vi "Lap Statistics.vi"   [LabVIEW 2014]
uses:
  <vilib>/Platform/TimedLoop/XDataNode/timing_clust.ctl
  <vilib>/Platform/TimedLoop/XDataNode/nitl_modes.ctl
  <vilib>/Platform/TimedLoop/XDataNode/wakeup.ctl
  Lap Statistics.ctl
  <vilib>/FPGAPlugInAG/sbRIO-9626/niLvFpga_Open_sbRIO-9626.vi
  <vilib>/rvi/interface/common/dynamic/niFpgaDynamicAddResources.vi
  Formula Hybrid 2012 r1/Global Data.vi
  <vilib>/Utility/error.llb/Error Cluster From Error Code.vi
  <vilib>/rvi/errors/niLvFpgaAdjustHostInterfaceError.vi
  <vilib>/Platform/TimedLoop/XDataNode/XDataNode.xnode
  <vilib>/rvi/interface/nirviOpenFPGA/nirviOpenFPGA.xnode
  FPGA Bitfiles/FormulaElectric2_FPGATarget_FPGA_8a5J0mMac2U.lvbitx
  <vilib>/rvi/interface/nirviReadWriteControl/nirviReadWriteControl.xnode
  <vilib>/Platform/TimedLoop/XDataNode/XDNodeRunTimeDep.lvlib
  NiFpgaLv.dll
  <vilib>/rvi/interface/Simulation/niFpgaSimulationCallBeginRW.vi
types:
  T1 = typedef "XDNodeRunTimeDep.lvlib/timing_clust.ctl" = cluster{"Expected End [f-1]":u64, "Actual End [f-1]":u64, "Finished Late? [f-1]":bool, "Expected End [i-1]":u64, "Actual End [i-1]":u64, "Finished Late? [i-1]":bool, "Expected Start [i]":u64, "Actual Start [i]":u64, "Expected Start [f]":u64, "Actual Start [f]":u64, "Source Name":string, "Structure Name":string, "Period":i64, "Deadline":i64, "Offset":i64, "Start":i64, "Priority":i32, "Timeout":i32, "Mode":T2, "Wakeup Reason":T3, "Error":errorcluster, "Source Type":string, "Secondary Source Type":string, "Global End Time":u64, "Global Start Time":u64, "Frame Duration":u64, "Iteration Duration":u64, "Assigned CPU":i32, "I/O Scan Engine Mode":u32}
  T2 = typedef "XDNodeRunTimeDep.lvlib/nitl_modes.ctl" = enum32{"No Change", "Process missed periods, maintain original phase", "Discard missed periods, maintain original phase", "Process missed periods, ignore original phase", "Discard missed periods, ignore original phase"}
  T3 = typedef "XDNodeRunTimeDep.lvlib/wakeup.ctl" = enum32{"Normal", "Aborted", "Asynchronous wakeup", "Timing source error", "Timed loop error", "Timeout"}
  T4 = typedef "Lap Statistics.ctl" = cluster{"rBrakeBalLast":dbl}
  T5 = cluster{"Accel X":dbl, "Accel Y":dbl, "Accel Z":dbl, "Gyro X":dbl, "Gyro Y":dbl, "Gyro Z":dbl}
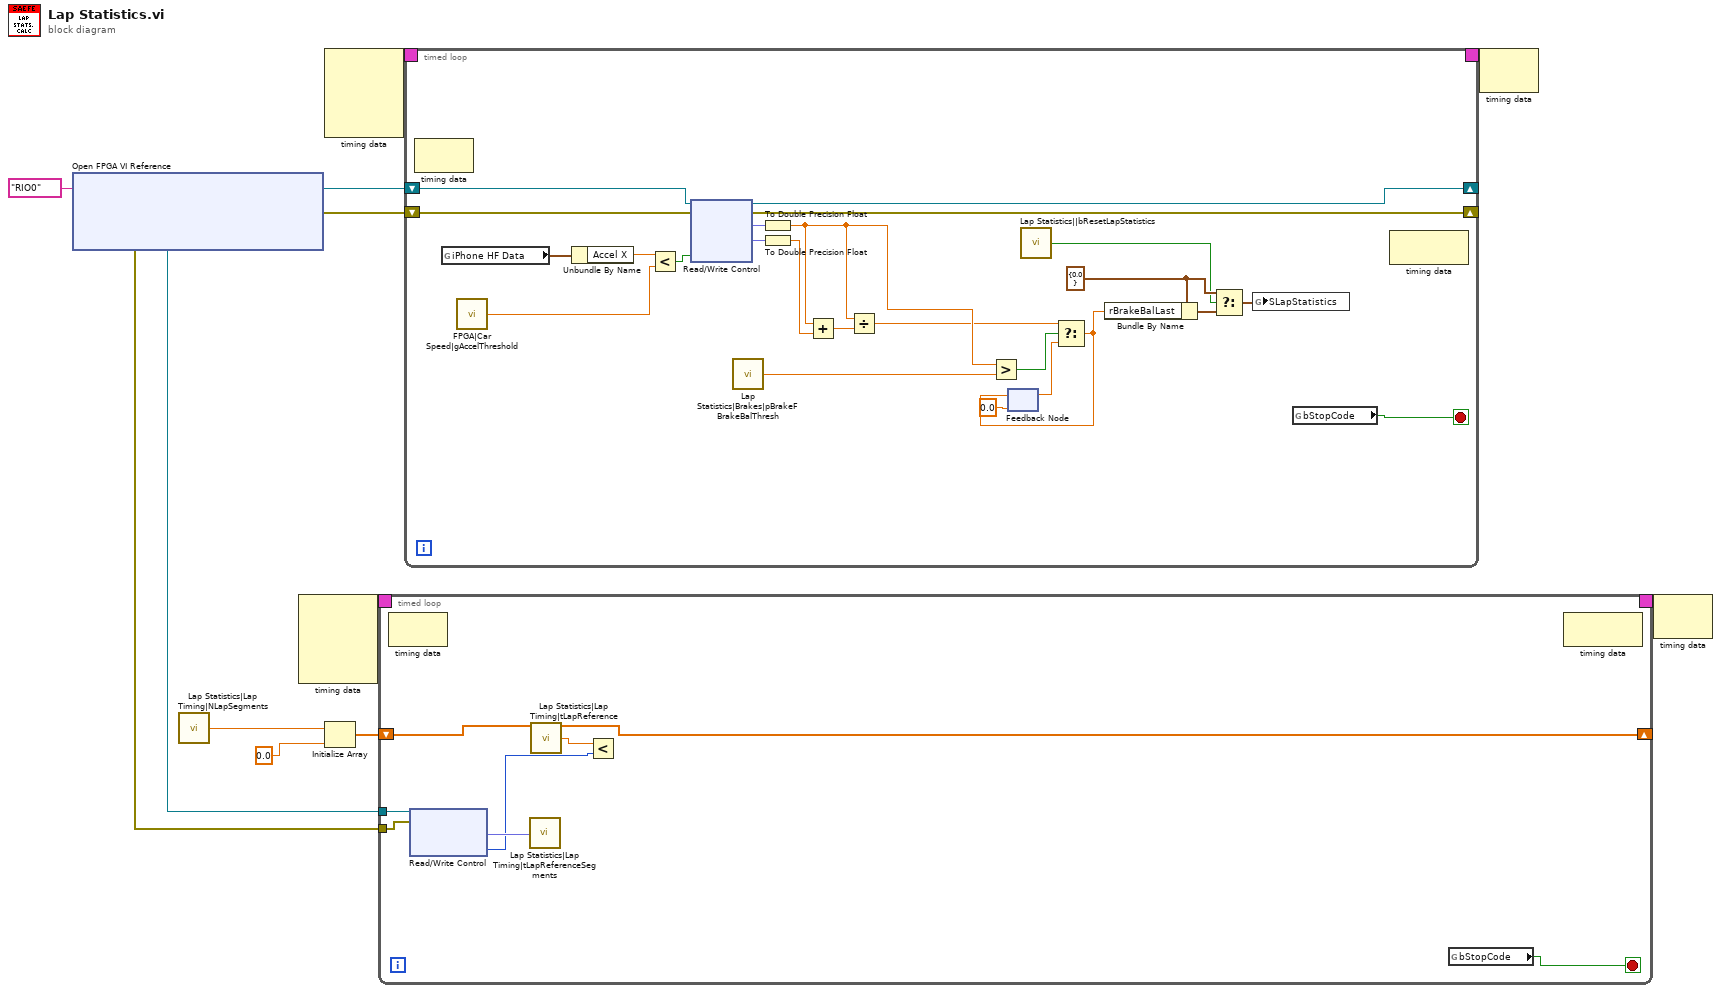
[diagram p0: block diagram]
diagram:
  n1 = xnode "Open FPGA VI Reference"("resource name"=tag "RIO0") -> ("FPGA VI Reference Out"=w5:refnum<k20>, "error out"=w4:errorcluster)  [unwired: 1 in]
  n2 = call "Lap Statistics|Lap Timing|NLapSegments"() -> ("Value"=w3:sgl)
  n3 = node-c288() -> (w7:T1)  [unwired: 4 in]
  n4 = node-c288() -> (w10:T1)  [unwired: 4 in]
  n5 = Initialize Array(w3, sgl 0.0) -> (w2:sgl[])
  n6 = timed-loop {
    timing: w7 -> [_]
    timing-out: [_] -> w6
    tunnel: w5 -> [w15]
    tunnel: w4 -> [w16]
    shift-right: [w11] -> _
    shift-left: w2 -> [w11]
    stop <- w17 stop-if-true
    n7 = node-c288() -> ()  [unwired: 1 in, 1 out]
    n8 = xnode "Read/Write Control"("FPGA VI Reference In"=w15, "error in"=w16) -> ("sLap"=w14:fxp<+,32,12>, "tFastestLap"=w12:u32)  [unwired: 2 out]
    n9 = call "Lap Statistics|Lap Timing|tLapReferenceSegments"("X Index"=w14) -> ()  [unwired: 1 out]
    n10 = call "Lap Statistics|Lap Timing|tLapReference"() -> ("Value"=w13:sgl)
    n11 = Less?(x=w13, y=w12) -> ()  [unwired: 1 out]
    n12 = global read "Global Data.vi" "bStopCode"() -> (w17:bool)
    n13 = node-c288() -> ()  [unwired: 1 in, 1 out]
  }
  n14 = timed-loop {
    timing: w10 -> [_]
    timing-out: [_] -> w9
    shift-right: [w41] -> _
    shift-left: w5 -> [w43]
    shift-right: [w40] -> _
    shift-left: w4 -> [w42]
    stop <- w39 stop-if-true
    w25 = T4 {"rBrakeBalLast"=0.0} ("Lap Statistics")
    n15 = node-c288() -> ()  [unwired: 1 in, 1 out]
    n16 = global read "Global Data.vi" "iPhone HF Data"() -> (w23:T5)
    n17 = call "FPGA|Car Speed|gAccelThreshold"() -> ("Value"=w20:sgl)
    n18 = Unbundle By Name(w23) -> ("Accel X"=w22:dbl)
    n19 = Less?(x=w22, y=w20) -> (x < y?=w21:bool)
    n20 = xnode "Read/Write Control"("FPGA VI Reference In"=w43, "error in"=w42, "bAccel"=w21) -> ("FPGA VI Reference Out"=w41:refnum<k20>, "error out"=w40:errorcluster, "pBrakeF"=w38:fxp<+,26,13>, "pBrakeR"=w37:fxp<+,26,13>)
    n21 = call "Lap Statistics|Brakes|pBrakeFBrakeBalThresh"() -> ("Value"=w33:sgl)
    n22 = To Double Precision Float(number=w38) -> (double precision float=w34:dbl)
    n23 = To Double Precision Float(number=w37) -> (double precision float=w36:dbl)
    n24 = Add(x=w34, y=w36) -> (x+y=w35:dbl)
    n25 = Divide(x=w34, y=w35) -> (x/y=w29:dbl)
    n26 = Greater?(x=w34, y=w33) -> (0:w31:bool)
    n27 = feedback #1(0.0) -> (w30:dbl)
    n28 = call "Lap Statistics||bResetLapStatistics"() -> ("Value"=w24:bool)
    n29 = Select(t=w29, s=w31, f=w30) -> (s? t:f=w28:dbl)
    n30 = feedback-in #1(w28) -> ()
    n31 = Bundle By Name(cluster=w25, "rBrakeBalLast"=w28) -> (w27:T4)
    n32 = Select(t=w25, s=w24, f=w27) -> (s? t:f=w26:T4)
    n33 = global write "Global Data.vi" "SLapStatistics"(w26) -> ()
    n34 = global read "Global Data.vi" "bStopCode"() -> (w39:bool)
    n35 = node-c288() -> ()  [unwired: 1 in, 1 out]
  }
  n36 = node-c288(w9) -> ()  [unwired: 1 out]
  n37 = node-c288(w6) -> ()  [unwired: 1 out]
